vi "rsidr_core_global.vi"() -> ()   [LabVIEW 2015, in "Rohde&Schwarz CMXP NR FR2 Measurement.lvlib"] (continued)
Available Repeated Capabilities:\ninstance: i0, i1, i2, i3, i4, i5, i6, i7, i8, i9, i10, i11, i12, i13, i14, i15, i16, i17, i18, i19, i20, i21, i22, i23, i24, i25, i26, i27, i28, i29, i30, i31, i32\r\n\nRemote-control command(s):\nCONFigure:NRMMw:MEAS<i>:MEValuation:LIMit:QAM64:EVMagnitude"}, {"Level"=5, "Class Only"=FALSE, "Identifier"="RSCMXPNRFR2M_ATTR_MULTI_EVAL_MEASUREMENT_LIMIT_QAM256_EVM", "Descriptive Name"="Multi Eval Measurement Limit QAM256 EVM", "Data Type"=enum."RawString", "Command"="CONF:NRMM:MEAS{instance}:MEV:LIM:QAM256:EVM", "Access"=enum."Read/Write", "Range Table"="", "Read Callback"="", "Write Callback"="", "Range Callback"="", "Check Callback"="", "Rngtable Callback"="", "Coerce Callback"="", "Supported Models"="", "Instrument Options"="", "Check Status Callback"="", "Flags"=0, "Help"="Defines upper limits for the RMS and peak values of the error vector magnitude (EVM) for QAM256.\n\nSyntax:\nCONFigure:NRMMw:MEAS<i>:MEValuation:LIMit:QAM256:EVMagnitude <RMS>, <Peak>\n\n<RMS>\nnumeric | ON | OFF\nValid Values:\n0 % to 100 %\nOFF\nON\n  \n<Peak>\nnumeric | ON | OFF\nValid Values:\n0 % to 100 %\nOFF\nON\n\nAvailable Repeated Capabilities:\ninstance: i0, i1, i2, i3, i4, i5, i6, i7, i8, i9, i10, i11, i12, i13, i14, i15, i16, i17, i18, i19, i20, i21, i22, i23, i24, i25, i26, i27, i28, i29, i30, i31, i32\r\n\nRemote-control command(s):\nCONFigure:NRMMw:MEAS<i>:MEValuation:LIMit:QAM256:EVMagnitude"}, {"Level"=5, "Class Only"=FALSE, "Identifier"="RSCMXPNRFR2M_ATTR_MULTI_EVAL_MEASUREMENT_LIMIT_QAM16_MERR", "Descriptive Name"="Multi Eval Measurement Limit QAM16 MERR", "Data Type"=enum."RawString", "Command"="CONF:NRMM:MEAS{instance}:MEV:LIM:QAM16:MERR", "Access"=enum."Read/Write", "Range Table"="", "Read Callback"="", "Write Callback"="", "Range Callback"="", "Check Callback"="", "Rngtable Callback"="", "Coerce Callback"="", "Supported Models"="", "Instrument Options"="", "Check Status Callback"="", "Flags"=0, "Help"="Defines upper limits for the RMS and peak values of the magnitude error (MERR)  for QAM16.\n\nSyntax:\nCONFigure:NRMMw:MEAS<i>:MEValuation:LIMit:QAM16:MERRor <RMS>, <Peak>\n\n<RMS>\nnumeric | ON | OFF\nValid Values:\n0 % to 100 %\nOFF\nON\n  \n<Peak>\nnumeric | ON | OFF\nValid Values:\n0 % to 100 %\nOFF\nON\n\nAvailable Repeated Capabilities:\ninstance: i0, i1, i2, i3, i4, i5, i6, i7, i8, i9, i10, i11, i12, i13, i14, i15, i16, i17, i18, i19, i20, i21, i22, i23, i24, i25, i26, i27, i28, i29, i30, i31, i32\r\n\nRemote-control command(s):\nCONFigure:NRMMw:MEAS<i>:MEValuation:LIMit:QAM16:MERRor"}, {"Level"=5, "Class Only"=FALSE, "Identifier"="RSCMXPNRFR2M_ATTR_MULTI_EVAL_MEASUREMENT_LIMIT_QAM64_MERR", "Descriptive Name"="Multi Eval Measurement Limit QAM64 MERR", "Data Type"=enum."RawString", "Command"="CONF:NRMM:MEAS{instance}:MEV:LIM:QAM64:MERR", "Access"=enum."Read/Write", "Range Table"="", "Read Callback"="", "Write Callback"="", "Range Callback"="", "Check Callback"="", "Rngtable Callback"="", "Coerce Callback"="", "Supported Models"="", "Instrument Options"="", "Check Status Callback"="", "Flags"=0, "Help"="Defines upper limits for the RMS and peak values of the magnitude error (MERR)  for QAM64.\n\nSyntax:\nCONFigure:NRMMw:MEAS<i>:MEValuation:LIMit:QAM64:MERRor <RMS>, <Peak>\n\n<RMS>\nnumeric | ON | OFF\nValid Values:\n0 % to 100 %\nOFF\nON\n  \n<Peak>\nnumeric | ON | OFF\nValid Values:\n0 % to 100 %\nOFF\nON\n\nAvailable Repeated Capabilities:\ninstance: i0, i1, i2, i3, i4, i5, i6, i7, i8, i9, i10, i11, i12, i13, i14, i15, i16, i17, i18, i19, i20, i21, i22, i23, i24, i25, i26, i27, i28, i29, i30, i31, i32\r\n\nRemote-control command(s):\nCONFigure:NRMMw:MEAS<i>:MEValuation:LIMit:QAM64:MERRor"}, {"Level"=5, "Class Only"=FALSE, "Identifier"="RSCMXPNRFR2M_ATTR_MULTI_EVAL_MEASUREMENT_LIMIT_QAM256_MERR", "Descriptive Name"="Multi Eval Measurement Limit QAM256 MERR", "Data Type"=enum."RawString", "Command"="CONF:NRMM:MEAS{instance}:MEV:LIM:QAM256:MERR", "Access"=enum."Read/Write", "Range Table"="", "Read Callback"="", "Write Callback"="", "Range Callback"="", "Check Callback"="", "Rngtable Callback"="", "Coerce Callback"="", "Supported Models"="", "Instrument Options"="", "Check Status Callback"="", "Flags"=0, "Help"="Defines upper limits for the RMS and peak values of the magnitude error (MERR)  for QAM256.\n\nSyntax:\nCONFigure:NRMMw:MEAS<i>:MEValuation:LIMit:QAM256:MERRor <RMS>, <Peak>\n\n<RMS>\nnumeric | ON | OFF\nValid Values:\n0 % to 100 %\nOFF\nON\n  \n<Peak>\nnumeric | ON | OFF\nValid Values:\n0 % to 100 %\nOFF\nON\n\nAvailable Repeated Capabilities:\ninstance: i0, i1, i2, i3, i4, i5, i6, i7, i8, i9, i10, i11, i12, i13, i14, i15, i16, i17, i18, i19, i20, i21, i22, i23, i24, i25, i26, i27, i28, i29, i30, i31, i32\r\n\nRemote-control command(s):\nCONFigure:NRMMw:MEAS<i>:MEValuation:LIMit:QAM256:MERRor"}, {"Level"=5, "Class Only"=FALSE, "Identifier"="RSCMXPNRFR2M_ATTR_MULTI_EVAL_MEASUREMENT_LIMIT_QAM16_PERR", "Descriptive Name"="Multi Eval Measurement Limit QAM16 PERR", "Data Type"=enum."RawString", "Command"="CONF:NRMM:MEAS{instance}:MEV:LIM:QAM16:PERR", "Access"=enum."Read/Write", "Range Table"="", "Read Callback"="", "Write Callback"="", "Range Callback"="", "Check Callback"="", "Rngtable Callback"="", "Coerce Callback"="", "Supported Models"="", "Instrument Options"="", "Check Status Callback"="", "Flags"=0, "Help"="Defines upper limits for the RMS and peak values of the phase error (PERR)  for QAM16.\n\nSyntax:\nCONFigure:NRMMw:MEAS<i>:MEValuation:LIMit:QAM16:PERRor <RMS>, <Peak>\n\n<RMS>\nnumeric | ON | OFF\nValid Values:\n0 % to 100 %\nOFF\nON\n  \n<Peak>\nnumeric | ON | OFF\nValid Values:\n0 % to 100 %\nOFF\nON\n\nAvailable Repeated Capabilities:\ninstance: i0, i1, i2, i3, i4, i5, i6, i7, i8, i9, i10, i11, i12, i13, i14, i15, i16, i17, i18, i19, i20, i21, i22, i23, i24, i25, i26, i27, i28, i29, i30, i31, i32\r\n\nRemote-control command(s):\nCONFigure:NRMMw:MEAS<i>:MEValuation:LIMit:QAM16:PERRor"}, {"Level"=5, "Class Only"=FALSE, "Identifier"="RSCMXPNRFR2M_ATTR_MULTI_EVAL_MEASUREMENT_LIMIT_QAM64_PERR", "Descriptive Name"="Multi Eval Measurement Limit QAM64 PERR", "Data Type"=enum."RawString", "Command"="CONF:NRMM:MEAS{instance}:MEV:LIM:QAM64:PERR", "Access"=enum."Read/Write", "Range Table"="", "Read Callback"="", "Write Callback"="", "Range Callback"="", "Check Callback"="", "Rngtable Callback"="", "Coerce Callback"="", "Supported Models"="", "Instrument Options"="", "Check Status Callback"="", "Flags"=0, "Help"="Defines upper limits for the RMS and peak values of the phase error (PERR)  for QAM64.\n\nSyntax:\nCONFigure:NRMMw:MEAS<i>:MEValuation:LIMit:QAM64:PERRor <RMS>, <Peak>\n\n<RMS>\nnumeric | ON | OFF\nValid Values:\n0 % to 100 %\nOFF\nON\n  \n<Peak>\nnumeric | ON | OFF\nValid Values:\n0 % to 100 %\nOFF\nON\n\nAvailable Repeated Capabilities:\ninstance: i0, i1, i2, i3, i4, i5, i6, i7, i8, i9, i10, i11, i12, i13, i14, i15, i16, i17, i18, i19, i20, i21, i22, i23, i24, i25, i26, i27, i28, i29, i30, i31, i32\r\n\nRemote-control command(s):\nCONFigure:NRMMw:MEAS<i>:MEValuation:LIMit:QAM64:PERRor"}, {"Level"=5, "Class Only"=FALSE, "Identifier"="RSCMXPNRFR2M_ATTR_MULTI_EVAL_MEASUREMENT_LIMIT_QAM256_PERR", "Descriptive Name"="Multi Eval Measurement Limit QAM256 PERR", "Data Type"=enum."RawString", "Command"="CONF:NRMM:MEAS{instance}:MEV:LIM:QAM256:PERR", "Access"=enum."Read/Write", "Range Table"="", "Read Callback"="", "Write Callback"="", "Range Callback"="", "Check Callback"="", "Rngtable Callback"="", "Coerce Callback"="", "Supported Models"="", "Instrument Options"="", "Check Status Callback"="", "Flags"=0, "Help"="Defines upper limits for the RMS and peak values of the phase error (PERR)  for QAM256.\n\nSyntax:\nCONFigure:NRMMw:MEAS<i>:MEValuation:LIMit:QAM256:PERRor <RMS>, <Peak>\n\n<RMS>\nnumeric | ON | OFF\nValid Values:\n0 % to 100 %\nOFF\nON\n  \n<Peak>\nnumeric | ON | OFF\nValid Values:\n0 % to 100 %\nOFF\nON\n\nAvailable Repeated Capabilities:\ninstance: i0, i1, i2, i3, i4, i5, i6, i7, i8, i9, i10, i11, i12, i13, i14, i15, i16, i17, i18, i19, i20, i21, i22, i23, i24, i25, i26, i27, i28, i29, i30, i31, i32\r\n\nRemote-control command(s):\nCONFigure:NRMMw:MEAS<i>:MEValuation:LIMit:QAM256:PERRor"}, {"Level"=5, "Class Only"=FALSE, "Identifier"="RSCMXPNRFR2M_ATTR_MULTI_EVAL_MEASUREMENT_LIMIT_QAM16_FERR", "Descriptive Name"="Multi Eval Measurement Limit QAM16 FERR", "Data Type"=enum."RawString", "Command"="CONF:NRMM:MEAS{instance}:MEV:LIM:QAM16:FERR", "Access"=enum."Read/Write", "Range Table"="", "Read Callback"="", "Write Callback"="", "Range Callback"="", "Check Callback"="", "Rngtable Callback"="", "Coerce Callback"="", "Supported Models"="", "Instrument Options"="", "Check Status Callback"="", "Flags"=0, "Help"="Defines an upper limit for the carrier frequency error.\n\nSyntax:\nCONFigure:NRMMw:MEAS<i>:MEValuation:LIMit:QAM16:FERRor <FrequencyError>\n\n<FrequencyError>\nnumeric | ON | OFF\nValid Values:\n0 to 1 ppm\nOFF\nON\n\nAvailable Repeated Capabilities:\ninstance: i0, i1, i2, i3, i4, i5, i6, i7, i8, i9, i10, i11, i12, i13, i14, i15, i16, i17, i18, i19, i20, i21, i22, i23, i24, i25, i26, i27, i28, i29, i30, i31, i32\r\n\nRemote-control command(s):\nCONFigure:NRMMw:MEAS<i>:MEValuation:LIMit:QAM16:FERRor"}, {"Level"=5, "Class Only"=FALSE, "Identifier"="RSCMXPNRFR2M_ATTR_MULTI_EVAL_MEASUREMENT_LIMIT_QAM64_FERR", "Descriptive Name"="Multi Eval Measurement Limit QAM64 FERR", "Data Type"=enum."RawString", "Command"="CONF:NRMM:MEAS{instance}:MEV:LIM:QAM64:FERR", "Access"=enum."Read/Write", "Range Table"="", "Read Callback"="", "Write Callback"="", "Range Callback"="", "Check Callback"="", "Rngtable Callback"="", "Coerce Callback"="", "Supported Models"="", "Instrument Options"="", "Check Status Callback"="", "Flags"=0, "Help"="Defines an upper limit for the carrier frequency error.\n\nSyntax:\nCONFigure:NRMMw:MEAS<i>:MEValuation:LIMit:QAM64:FERRor <FrequencyError>\n\n<FrequencyError>\nnumeric | ON | OFF\nValid Values:\n0 to 1 ppm\nOFF\nON\n\nAvailable Repeated Capabilities:\ninstance: i0, i1, i2, i3, i4, i5, i6, i7, i8, i9, i10, i11, i12, i13, i14, i15, i16, i17, i18, i19, i20, i21, i22, i23, i24, i25, i26, i27, i28, i29, i30, i31, i32\r\n\nRemote-control command(s):\nCONFigure:NRMMw:MEAS<i>:MEValuation:LIMit:QAM64:FERRor"}, {"Level"=5, "Class Only"=FALSE, "Identifier"="RSCMXPNRFR2M_ATTR_MULTI_EVAL_MEASUREMENT_LIMIT_QAM256_FERR", "Descriptive Name"="Multi Eval Measurement Limit QAM256 FERR", "Data Type"=enum."RawString", "Command"="CONF:NRMM:MEAS{instance}:MEV:LIM:QAM256:FERR", "Access"=enum."Read/Write", "Range Table"="", "Read Callback"="", "Write Callback"="", "Range Callback"="", "Check Callback"="", "Rngtable Callback"="", "Coerce Callback"="", "Supported Models"="", "Instrument Options"="", "Check Status Callback"="", "Flags"=0, "Help"="Defines an upper limit for the carrier frequency error.\n\nSyntax:\nCONFigure:NRMMw:MEAS<i>:MEValuation:LIMit:QAM256:FERRor <FrequencyError>\n\n<FrequencyError>\nnumeric | ON | OFF\nValid Values:\n0 to 1 ppm\nOFF\nON\n\nAvailable Repeated Capabilities:\ninstance: i0, i1, i2, i3, i4, i5, i6, i7, i8, i9, i10, i11, i12, i13, i14, i15, i16, i17, i18, i19, i20, i21, i22, i23, i24, i25, i26, i27, i28, i29, i30, i31, i32\r\n\nRemote-control command(s):\nCONFigure:NRMMw:MEAS<i>:MEValuation:LIMit:QAM256:FERRor"}, {"Level"=5, "Class Only"=FALSE, "Identifier"="RSCMXPNRFR2M_ATTR_MULTI_EVAL_MEASUREMENT_LIMIT_QAM16_IQ_OFFSET", "Descriptive Name"="Multi Eval Measurement Limit QAM16 IQ Offset", "Data Type"=enum."RawString", "Command"="CONF:NRMM:MEAS{instance}:MEV:LIM:QAM16:IQOF", "Access"=enum."Read/Write", "Range Table"="", "Read Callback"="", "Write Callback"="", "Range Callback"="", "Check Callback"="", "Rngtable Callback"="", "Coerce Callback"="", "Supported Models"="", "Instrument Options"="", "Check Status Callback"="", "Flags"=0, "Help"="Defines upper limits for the I/Q origin offset (QAM16 modulation). Two different I/Q origin offset limits can be set for two TX power ranges.\n\nSyntax:\nCONFigure:NRMMw:MEAS<i>:MEValuation:LIMit:QAM16:IQOFfset <Enable>, <Offset0>, <Offset1>\n\n<Enable>\nValid Values:\nOFF: disables the limit check\nON: enables the limit check\n\n<Offset0>\nI/Q origin offset limit for TX power > 0 dBm\nnumeric\nValid Values: -256 dBc to 256 dBc\n\n<Offset1>\nI/Q origin offset limit for TX power  0 dBm\nnumeric\nValid Values: -256 dBc to 256 dBc\n\nAvailable Repeated Capabilities:\ninstance: i0, i1, i2, i3, i4, i5, i6, i7, i8, i9, i10, i11, i12, i13, i14, i15, i16, i17, i18, i19, i20, i21, i22, i23, i24, i25, i26, i27, i28, i29, i30, i31, i32\r\n\nRemote-control command(s):\nCONFigure:NRMMw:MEAS<i>:MEValuation:LIMit:QAM16:IQOFfset"}, {"Level"=5, "Class Only"=FALSE, "Identifier"="RSCMXPNRFR2M_ATTR_MULTI_EVAL_MEASUREMENT_LIMIT_QAM64_IQ_OFFSET", "Descriptive Name"="Multi Eval Measurement Limit QAM64 IQ Offset", "Data Type"=enum."RawString", "Command"="CONF:NRMM:MEAS{instance}:MEV:LIM:QAM64:IQOF", "Access"=enum."Read/Write", "Range Table"="", "Read Callback"="", "Write Callback"="", "Range Callback"="", "Check Callback"="", "Rngtable Callback"="", "Coerce Callback"="", "Supported Models"="", "Instrument Options"="", "Check Status Callback"="", "Flags"=0, "Help"="Defines upper limits for the I/Q origin offset (QAM64 modulation). Two different I/Q origin offset limits can be set for two TX power ranges.\n\nSyntax:\nCONFigure:NRMMw:MEAS<i>:MEValuation:LIMit:QAM64:IQOFfset <Enable>, <Offset0>, <Offset1>\n\n<Enable>\nValid Values:\nOFF: disables the limit check\nON: enables the limit check\n\n<Offset0>\nI/Q origin offset limit for TX power > 0 dBm\nnumeric\nValid Values: -256 dBc to 256 dBc\n\n<Offset1>\nI/Q origin offset limit for TX power  0 dBm\nnumeric\nValid Values: -256 dBc to 256 dBc\n\nAvailable Repeated Capabilities:\ninstance: i0, i1, i2, i3, i4, i5, i6, i7, i8, i9, i10, i11, i12, i13, i14, i15, i16, i17, i18, i19, i20, i21, i22, i23, i24, i25, i26, i27, i28, i29, i30, i31, i32\r\n\nRemote-control command(s):\nCONFigure:NRMMw:MEAS<i>:MEValuation:LIMit:QAM64:IQOFfset"}, {"Level"=5, "Class Only"=FALSE, "Identifier"="RSCMXPNRFR2M_ATTR_MULTI_EVAL_MEASUREMENT_LIMIT_QAM256_IQ_OFFSET", "Descriptive Name"="Multi Eval Measurement Limit QAM256 IQ Offset", "Data Type"=enum."RawString", "Command"="CONF:NRMM:MEAS{instance}:MEV:LIM:QAM256:IQOF", "Access"=enum."Read/Write", "Range Table"="", "Read Callback"="", "Write Callback"="", "Range Callback"="", "Check Callback"="", "Rngtable Callback"="", "Coerce Callback"="", "Supported Models"="", "Instrument Options"="", "Check Status Callback"="", "Flags"=0, "Help"="Defines upper limits for the I/Q origin offset (QAM256 modulation). Two different I/Q origin offset limits can be set for two TX power ranges.\n\nSyntax:\nCONFigure:NRMMw:MEAS<i>:MEValuation:LIMit:QAM256:IQOFfset <Enable>, <Offset0>, <Offset1>\n\n<Enable>\nValid Values:\nOFF: disables the limit check\nON: enables the limit check\n\n<Offset0>\nI/Q origin offset limit for TX power > 0 dBm\nnumeric\nValid Values: -256 dBc to 256 dBc\n\n<Offset1>\nI/Q origin offset limit for TX power  0 dBm\nnumeric\nValid Values: -256 dBc to 256 dBc\n\nAvailable Repeated Capabilities:\ninstance: i0, i1, i2, i3, i4, i5, i6, i7, i8, i9, i10, i11, i12, i13, i14, i15, i16, i17, i18, i19, i20, i21, i22, i23, i24, i25, i26, i27, i28, i29, i30, i31, i32\r\n\nRemote-control command(s):\nCONFigure:NRMMw:MEAS<i>:MEValuation:LIMit:QAM256:IQOFfset"}, {"Level"=5, "Class Only"=FALSE, "Identifier"="RSCMXPNRFR2M_ATTR_MULTI_EVAL_MEASUREMENT_LIMIT_QAM16_INBAND_EMISSION", "Descriptive Name"="Multi Eval Measurement Limit QAM16 Inband Emission", "Data Type"=enum."RawString", "Command"="CONF:NRMM:MEAS{instance}:MEV:LIM:QAM16:IBE", "Access"=enum."Read/Write", "Range Table"="", "Read Callback"="", "Write Callback"="", "Range Callback"="", "Check Callback"="", "Rngtable Callback"="", "Coerce Callback"="", "Supported Models"="", "Instrument Options"="", "Check Status Callback"="", "Flags"=0, "Help"="Defines parameters used for calculation of an upper limit for the inband emission (QAM16 modulation).\n\nSyntax:\nCONFigure:NRMMw:MEAS<i>:MEValuation:LIMit:QAM16:IQOFfset <Enable>, <Offset0>, <Offset1>\n\n<Enable>\nValid Values:\nOFF: disables the limit check\nON: enables the limit check\n\n<Minimum>\nnumeric\nValid Values: -256 dB to 256 dB\n\n<EVM>\nnumeric\nValid Values: 0 % to 100 %\n\n<RBPower>\nnumeric\nValid Values: -256 dBm to 256 dBm\n\n<IQImageLesser>\nIQ image for low TX power range\nnumeric\nValid Values: -256 dB to 256 dB\n \n<IQImageGreater>\nIQ image for high TX power range\nnumeric\nValid Values: -256 dB  to  256 dB\n\nAvailable Repeated Capabilities:\ninstance: i0, i1, i2, i3, i4, i5, i6, i7, i8, i9, i10, i11, i12, i13, i14, i15, i16, i17, i18, i19, i20, i21, i22, i23, i24, i25, i26, i27, i28, i29, i30, i31, i32\r\n\nRemote-control command(s):\nCONFigure:NRMMw:MEAS<i>:MEValuation:LIMit:QAM16:IBE"}, {"Level"=5, "Class Only"=FALSE, "Identifier"="RSCMXPNRFR2M_ATTR_MULTI_EVAL_MEASUREMENT_LIMIT_QAM64_INBAND_EMISSION", "Descriptive Name"="Multi Eval Measurement Limit QAM64 Inband Emission", "Data Type"=enum."RawString", "Command"="CONF:NRMM:MEAS{instance}:MEV:LIM:QAM64:IBE", "Access"=enum."Read/Write", "Range Table"="", "Read Callback"="", "Write Callback"="", "Range Callback"="", "Check Callback"="", "Rngtable Callback"="", "Coerce Callback"="", "Supported Models"="", "Instrument Options"="", "Check Status Callback"="", "Flags"=0, "Help"="Defines parameters used for calculation of an upper limit for the inband emission (QAM64 modulation).\n\nSyntax:\nCONFigure:NRMMw:MEAS<i>:MEValuation:LIMit:QAM64:IQOFfset <Enable>, <Offset0>, <Offset1>\n\n<Enable>\nValid Values:\nOFF: disables the limit check\nON: enables the limit check\n\n<Minimum>\nnumeric\nValid Values: -256 dB to 256 dB\n\n<EVM>\nnumeric\nValid Values: 0 % to 100 %\n\n<RBPower>\nnumeric\nValid Values: -256 dBm to 256 dBm\n\n<IQImageLesser>\nIQ image for low TX power range\nnumeric\nValid Values: -256 dB to 256 dB\n \n<IQImageGreater>\nIQ image for high TX power range\nnumeric\nValid Values: -256 dB  to  256 dB\n\nAvailable Repeated Capabilities:\ninstance: i0, i1, i2, i3, i4, i5, i6, i7, i8, i9, i10, i11, i12, i13, i14, i15, i16, i17, i18, i19, i20, i21, i22, i23, i24, i25, i26, i27, i28, i29, i30, i31, i32\r\n\nRemote-control command(s):\nCONFigure:NRMMw:MEAS<i>:MEValuation:LIMit:QAM64:IBE"}, {"Level"=5, "Class Only"=FALSE, "Identifier"="RSCMXPNRFR2M_ATTR_MULTI_EVAL_MEASUREMENT_LIMIT_QAM256_INBAND_EMISSION", "Descriptive Name"="Multi Eval Measurement Limit QAM256 Inband Emission", "Data Type"=enum."RawString", "Command"="CONF:NRMM:MEAS{instance}:MEV:LIM:QAM256:IBE", "Access"=enum."Read/Write", "Range Table"="", "Read Callback"="", "Write Callback"="", "Range Callback"="", "Check Callback"="", "Rngtable Callback"="", "Coerce Callback"="", "Supported Models"="", "Instrument Options"="", "Check Status Callback"="", "Flags"=0, "Help"="Defines parameters used for calculation of an upper limit for the inband emission (QAM256 modulation).\n\nSyntax:\nCONFigure:NRMMw:MEAS<i>:MEValuation:LIMit:QAM256:IQOFfset <Enable>, <Offset0>, <Offset1>\n\n<Enable>\nValid Values:\nOFF: disables the limit check\nON: enables the limit check\n\n<Minimum>\nnumeric\nValid Values: -256 dB to 256 dB\n\n<EVM>\nnumeric\nValid Values: 0 % to 100 %\n\n<RBPower>\nnumeric\nValid Values: -256 dBm to 256 dBm\n\n<IQImageLesser>\nIQ image for low TX power range\nnumeric\nValid Values: -256 dB to 256 dB\n \n<IQImageGreater>\nIQ image for high TX power range\nnumeric\nValid Values: -256 dB  to  256 dB\n\nAvailable Repeated Capabilities:\ninstance: i0, i1, i2, i3, i4, i5, i6, i7, i8, i9, i10, i11, i12, i13, i14, i15, i16, i17, i18, i19, i20, i21, i22, i23, i24, i25, i26, i27, i28, i29, i30, i31, i32\r\n\nRemote-control command(s):\nCONFigure:NRMMw:MEAS<i>:MEValuation:LIMit:QAM256:IBE"}, {"Level"=5, "Class Only"=FALSE, "Identifier"="RSCMXPNRFR2M_ATTR_MULTI_EVAL_MEASUREMENT_LIMIT_QAM16_INBAND_EMISSION_IQ_OFFSET", "Descriptive Name"="Multi Eval Measurement Limit QAM16 Inband Emission IQ Offset", "Data Type"=enum."RawString", "Command"="CONF:NRMM:MEAS{instance}:MEV:LIM:QAM16:IBE:IQOF", "Access"=enum."Read/Write", "Range Table"="", "Read Callback"="", "Write Callback"="", "Range Callback"="", "Check Callback"="", "Rngtable Callback"="", "Coerce Callback"="", "Supported Models"="", "Instrument Options"="", "Check Status Callback"="", "Flags"=0, "Help"="Defines I/Q origin offset values used for calculation of an upper limit for the inband emission, for QAM16 modulation. Two different values can be set for two TX power ranges.\n\nSyntax:\nCONFigure:NRMMw:MEAS<i>:MEValuation:LIMit:QAM16:IBE:IQOFfset <Offset0>, <Offset1>\n\n<Offset0>\nI/Q origin offset limit for TX power > 0 dBm\nnumeric\nValid Values: -256 dBc to 256 dBc\n\n<Offset1>\nI/Q origin offset limit for TX power  0 dBm\nnumeric\nValid Values: -256 dBc to 256 dBc\n\nAvailable Repeated Capabilities:\ninstance: i0, i1, i2, i3, i4, i5, i6, i7, i8, i9, i10, i11, i12, i13, i14, i15, i16, i17, i18, i19, i20, i21, i22, i23, i24, i25, i26, i27, i28, i29, i30, i31, i32\r\n\nRemote-control command(s):\nCONFigure:NRMMw:MEAS<i>:MEValuation:LIMit:QAM16:IBE:IQOFfset"}, {"Level"=5, "Class Only"=FALSE, "Identifier"="RSCMXPNRFR2M_ATTR_MULTI_EVAL_MEASUREMENT_LIMIT_QAM64_INBAND_EMISSION_IQ_OFFSET", "Descriptive Name"="Multi Eval Measurement Limit QAM64 Inband Emission IQ Offset", "Data Type"=enum."RawString", "Command"="CONF:NRMM:MEAS{instance}:MEV:LIM:QAM64:IBE:IQOF", "Access"=enum."Read/Write", "Range Table"="", "Read Callback"="", "Write Callback"="", "Range Callback"="", "Check Callback"="", "Rngtable Callback"="", "Coerce Callback"="", "Supported Models"="", "Instrument Options"="", "Check Status Callback"="", "Flags"=0, "Help"="Defines I/Q origin offset values used for calculation of an upper limit for the inband emission, for QAM64 modulation. Two different values can be set for two TX power ranges.\n\nSyntax:\nCONFigure:NRMMw:MEAS<i>:MEValuation:LIMit:QAM64:IBE:IQOFfset <Offset0>, <Offset1>\n\n<Offset0>\nI/Q origin offset limit for TX power > 0 dBm\nnumeric\nValid Values: -256 dBc to 256 dBc\n\n<Offset1>\nI/Q origin offset limit for TX power  0 dBm\nnumeric\nValid Values: -256 dBc to 256 dBc\n\nAvailable Repeated Capabilities:\ninstance: i0, i1, i2, i3, i4, i5, i6, i7, i8, i9, i10, i11, i12, i13, i14, i15, i16, i17, i18, i19, i20, i21, i22, i23, i24, i25, i26, i27, i28, i29, i30, i31, i32\r\n\nRemote-control command(s):\nCONFigure:NRMMw:MEAS<i>:MEValuation:LIMit:QAM64:IBE:IQOFfset"}, {"Level"=5, "Class Only"=FALSE, "Identifier"="RSCMXPNRFR2M_ATTR_MULTI_EVAL_MEASUREMENT_LIMIT_QAM256_INBAND_EMISSION_IQ_OFFSET", "Descriptive Name"="Multi Eval Measurement Limit QAM256 Inband Emission IQ Offset", "Data Type"=enum."RawString", "Command"="CONF:NRMM:MEAS{instance}:MEV:LIM:QAM256:IBE:IQOF", "Access"=enum."Read/Write", "Range Table"="", "Read Callback"="", "Write Callback"="", "Range Callback"="", "Check Callback"="", "Rngtable Callback"="", "Coerce Callback"="", "Supported Models"="", "Instrument Options"="", "Check Status Callback"="", "Flags"=0, "Help"="Defines I/Q origin offset values used for calculation of an upper limit for the inband emission, for QAM256 modulation. Two different values can be set for two TX power ranges.\n\nSyntax:\nCONFigure:NRMMw:MEAS<i>:MEValuation:LIMit:QAM256:IBE:IQOFfset <Offset0>, <Offset1>\n\n<Offset0>\nI/Q origin offset limit for TX power > 0 dBm\nnumeric\nValid Values: -256 dBc to 256 dBc\n\n<Offset1>\nI/Q origin offset limit for TX power  0 dBm\nnumeric\nValid Values: -256 dBc to 256 dBc\n\nAvailable Repeated Capabilities:\ninstance: i0, i1, i2, i3, i4, i5, i6, i7, i8, i9, i10, i11, i12, i13, i14, i15, i16, i17, i18, i19, i20, i21, i22, i23, i24, i25, i26, i27, i28, i29, i30, i31, i32\r\n\nRemote-control command(s):\nCONFigure:NRMMw:MEAS<i>:MEValuation:LIMit:QAM256:IBE:IQOFfset"}, {"Level"=5, "Class Only"=FALSE, "Identifier"="RSCMXPNRFR2M_ATTR_MULTI_EVAL_MEASUREMENT_LIMIT_QAM16_EQUALIZER_SPECTRUM_FLATNESS", "Descriptive Name"="Multi Eval Measurement Limit QAM16 Equalizer Spectrum Flatness", "Data Type"=enum."RawString", "Command"="CONF:NRMM:MEAS{instance}:MEV:LIM:QAM16:ESFL", "Access"=enum."Read/Write", "Range Table"="", "Read Callback"="", "Write Callback"="", "Range Callback"="", "Check Callback"="", "Rngtable Callback"="", "Coerce Callback"="", "Supported Models"="", "Instrument Options"="", "Check Status Callback"="", "Flags"=0, "Help"="Defines limits for the equalizer spectrum flatness (QAM16 modulation).\n\nSyntax:\nCONFigure:NRMMw:MEAS<i>:MEValuation:LIMit:QAM16:IQOFfset <Enable>, <Offset0>, <Offset1>\n\n<Enable>\nValid Values:\nOFF: disables the limit check\nON: enables the limit check\n\n<Range1>\nUpper limit for max(range 1) - min(range 1)\nnumeric\nValid Values: -256 dBpp to 256 dBpp \n\n<Range2>\nUpper limit for max(range 2) - min(range 2)\nnumeric\nValid Values: -256 dBpp to 256 dBpp \n\n<Max1Min2>\nUpper limit for max(range 1) - min(range 2)\nnumeric\nValid Values: -256 dB to 256 dB \n\n<Max2Min1>\nUpper limit for max(range 2) - min(range 1)\nnumeric\nValid Values: -256 dB to 256 dB\n\nAvailable Repeated Capabilities:\ninstance: i0, i1, i2, i3, i4, i5, i6, i7, i8, i9, i10, i11, i12, i13, i14, i15, i16, i17, i18, i19, i20, i21, i22, i23, i24, i25, i26, i27, i28, i29, i30, i31, i32\r\n\nRemote-control command(s):\nCONFigure:NRMMw:MEAS<i>:MEValuation:LIMit:QAM16:ESFLatness"}, {"Level"=5, "Class Only"=FALSE, "Identifier"="RSCMXPNRFR2M_ATTR_MULTI_EVAL_MEASUREMENT_LIMIT_QAM64_EQUALIZER_SPECTRUM_FLATNESS", "Descriptive Name"="Multi Eval Measurement Limit QAM64 Equalizer Spectrum Flatness", "Data Type"=enum."RawString", "Command"="CONF:NRMM:MEAS{instance}:MEV:LIM:QAM64:ESFL", "Access"=enum."Read/Write", "Range Table"="", "Read Callback"="", "Write Callback"="", "Range Callback"="", "Check Callback"="", "Rngtable Callback"="", "Coerce Callback"="", "Supported Models"="", "Instrument Options"="", "Check Status Callback"="", "Flags"=0, "Help"="Defines limits for the equalizer spectrum flatness (QAM64 modulation).\n\nSyntax:\nCONFigure:NRMMw:MEAS<i>:MEValuation:LIMit:QAM64:IQOFfset <Enable>, <Offset0>, <Offset1>\n\n<Enable>\nValid Values:\nOFF: disables the limit check\nON: enables the limit check\n\n<Range1>\nUpper limit for max(range 1) - min(range 1)\nnumeric\nValid Values: -256 dBpp to 256 dBpp \n\n<Range2>\nUpper limit for max(range 2) - min(range 2)\nnumeric\nValid Values: -256 dBpp to 256 dBpp \n\n<Max1Min2>\nUpper limit for max(range 1) - min(range 2)\nnumeric\nValid Values: -256 dB to 256 dB \n\n<Max2Min1>\nUpper limit for max(range 2) - min(range 1)\nnumeric\nValid Values: -256 dB to 256 dB\n\nAvailable Repeated Capabilities:\ninstance: i0, i1, i2, i3, i4, i5, i6, i7, i8, i9, i10, i11, i12, i13, i14, i15, i16, i17, i18, i19, i20, i21, i22, i23, i24, i25, i26, i27, i28, i29, i30, i31, i32\r\n\nRemote-control command(s):\nCONFigure:NRMMw:MEAS<i>:MEValuation:LIMit:QAM64:ESFLatness"}, {"Level"=5, "Class Only"=FALSE, "Identifier"="RSCMXPNRFR2M_ATTR_MULTI_EVAL_MEASUREMENT_LIMIT_QAM256_EQUALIZER_SPECTRUM_FLATNESS", "Descriptive Name"="Multi Eval Measurement Limit QAM256 Equalizer Spectrum Flatness", "Data Type"=enum."RawString", "Command"="CONF:NRMM:MEAS{instance}:MEV:LIM:QAM256:ESFL", "Access"=enum."Read/Write", "Range Table"="", "Read Callback"="", "Write Callback"="", "Range Callback"="", "Check Callback"="", "Rngtable Callback"="", "Coerce Callback"="", "Supported Models"="", "Instrument Options"="", "Check Status Callback"="", "Flags"=0, "Help"="Defines limits for the equalizer spectrum flatness (QAM256 modulation).\n\nSyntax:\nCONFigure:NRMMw:MEAS<i>:MEValuation:LIMit:QAM256:IQOFfset <Enable>, <Offset0>, <Offset1>\n\n<Enable>\nValid Values:\nOFF: disables the limit check\nON: enables the limit check\n\n<Range1>\nUpper limit for max(range 1) - min(range 1)\nnumeric\nValid Values: -256 dBpp to 256 dBpp \n\n<Range2>\nUpper limit for max(range 2) - min(range 2)\nnumeric\nValid Values: -256 dBpp to 256 dBpp \n\n<Max1Min2>\nUpper limit for max(range 1) - min(range 2)\nnumeric\nValid Values: -256 dB to 256 dB \n\n<Max2Min1>\nUpper limit for max(range 2) - min(range 1)\nnumeric\nValid Values: -256 dB to 256 dB\n\nAvailable Repeated Capabilities:\ninstance: i0, i1, i2, i3, i4, i5, i6, i7, i8, i9, i10, i11, i12, i13, i14, i15, i16, i17, i18, i19, i20, i21, i22, i23, i24, i25, i26, i27, i28, i29, i30, i31, i32\r\n\nRemote-control command(s):\nCONFigure:NRMMw:MEAS<i>:MEValuation:LIMit:QAM256:ESFLatness"}, {"Level"=3, "Class Only"=TRUE, "Identifier"="", "Descriptive Name"="Spectrum", "Data Type"=enum."ViInt32", "Command"="", "Access"=enum."Read Only", "Range Table"="", "Read Callback"="", "Write Callback"="", "Range Callback"="", "Check Callback"="", "Rngtable Callback"="", "Coerce Callback"="", "Supported Models"="", "Instrument Options"="", "Check Status Callback"="", "Flags"=0, "Help"="Spectrum limits definition."}, {"Level"=4, "Class Only"=FALSE, "Identifier"="RSCMXPNRFR2M_ATTR_MULTI_EVAL_MEASUREMENT_LIMIT_OBW_ENABLED", "Descriptive Name"="Multi Eval Measurement Limit OBW Enabled", "Data Type"=enum."ViBoolean", "Command"="CONF:NRMM:MEAS{instance}:MEV:LIM:SEM:OBWL:CBAN{Bandwidth}", "Access"=enum."Write Only", "Range Table"="", "Read Callback"="", "Write Callback"="", "Range Callback"="", "Check Callback"="", "Rngtable Callback"="", "Coerce Callback"="", "Supported Models"="", "Instrument Options"="", "Check Status Callback"="", "Flags"=0, "Help"="Enables/disables an upper limit for the occupied bandwidth, depending on the channel bandwidth.\n\nAvailable Repeated Capabilities:\ninstance: i0, i1, i2, i3, i4, i5, i6, i7, i8, i9, i10, i11, i12, i13, i14, i15, i16, i17, i18, i19, i20, i21, i22, i23, i24, i25, i26, i27, i28, i29, i30, i31, i32\r\nBandwidth: BW50, BW100, BW200, BW400\r\n\nRemote-control command(s):\nCONFigure:NRMMw:MEAS<i>:MEValuation:LIMit:SEMask:OBWLimit:CBANdwidth<bw>"}, {"Level"=4, "Class Only"=FALSE, "Identifier"="RSCMXPNRFR2M_ATTR_MULTI_EVAL_MEASUREMENT_LIMIT_OBW", "Descriptive Name"="Multi Eval Measurement Limit OBW", "Data Type"=enum."ViReal64", "Command"="CONF:NRMM:MEAS{instance}:MEV:LIM:SEM:OBWL:CBAN{Bandwidth}", "Access"=enum."Read/Write", "Range Table"="rsCmxpNrFr2M_rngOBWLimit", "Read Callback"="", "Write Callback"="", "Range Callback"="", "Check Callback"="", "Rngtable Callback"="", "Coerce Callback"="", "Supported Models"="", "Instrument Options"="", "Check Status Callback"="", "Flags"=0, "Help"="Defines an upper limit for the occupied bandwidth, depending on the channel bandwidth.\n\nAvailable Repeated Capabilities:\ninstance: i0, i1, i2, i3, i4, i5, i6, i7, i8, i9, i10, i11, i12, i13, i14, i15, i16, i17, i18, i19, i20, i21, i22, i23, i24, i25, i26, i27, i28, i29, i30, i31, i32\r\nBandwidth: BW50, BW100, BW200, BW400\r\n\nRemote-control command(s):\nCONFigure:NRMMw:MEAS<i>:MEValuation:LIMit:SEMask:OBWLimit:CBANdwidth<bw>"}, {"Level"=4, "Class Only"=FALSE, "Identifier"="RSCMXPNRFR2M_ATTR_MULTI_EVAL_MEASUREMENT_LIMIT_EMISSION_MASK", "Descriptive Name"="Multi Eval Measurement Limit Emission Mask", "Data Type"=enum."RawString", "Command"="CONF:NRMM:MEAS{instance}:MEV:LIM:SEM:AREA{Area}:CBAN{Bandwidth}", "Access"=enum."Read/Write", "Range Table"="", "Read Callback"="", "Write Callback"="", "Range Callback"="", "Check Callback"="", "Rngtable Callback"="", "Coerce Callback"="", "Supported Models"="", "Instrument Options"="", "Check Status Callback"="", "Flags"=0, "Help"="Defines general requirements for the emission mask area number <area>. The activation state, the area borders, an upper limit and the resolution bandwidth must be specified.\nThe emission mask applies to the channel bandwidth <bw>.\n\nSyntax:\nCONFigure:NRMMw:MEAS<i>:MEValuation:LIMit:SEMask:AREA<area>:CBANdwidth<bw> <Enable>, <FrequencyStart>, <FrequencyEnd>, <Level>, <RBW>\n\n<bw>\nChannel bandwidth in MHz\nValid Values: 50, 100, 200, 400\n \n<area>\nNumber of the emission mask area\nValid Values: 1 to 12\n\n<Enable>\nValid Values:\nOFF: disables the check of these requirements\nON: enables the check of these requirements\n \n<FrequencyStart>\nStart frequency of the area, relative to the edges of the channel bandwidth\nnumeric\nValid Values: 0 MHz to 405 MHz (less, depending on <bw>) \n \n<FrequencyEnd>\nStop frequency of the area, relative to the edges of the channel bandwidth\nnumeric\nValid Values: 0 MHz to 405 MHz (less, depending on <bw>)\n\n<Level>\nUpper limit for the area\nnumeric\nValid Values: -256 dBm to 256 dBm\n\n<RBW>\nResolution bandwidth to be used for the area (1 MHz)\nValid Values: M1\n\nAvailable Repeated Capabilities:\ninstance: i0, i1, i2, i3, i4, i5, i6, i7, i8, i9, i10, i11, i12, i13, i14, i15, i16, i17, i18, i19, i20, i21, i22, i23, i24, i25, i26, i27, i28, i29, i30, i31, i32\r\nArea: a1, a2, a3, a4, a5, a6, a7, a8, a9, a10, a11, a12\r\nBandwidth: BW50, BW100, BW200, BW400\r\n\nRemote-control command(s):\nCONFigure:NRMMw:MEAS<i>:MEValuation:LIMit:SEMask:AREA<area>:CBANdwidth<bw>"}, {"Level"=4, "Class Only"=FALSE, "Identifier"="RSCMXPNRFR2M_ATTR_MULTI_EVAL_MEASUREMENT_LIMIT_EMISSION_MASK_TEST_TOLERANCE", "Descriptive Name"="Multi Eval Measurement Limit Emission Mask Test Tolerance", "Data Type"=enum."RawString", "Command"="CONF:NRMM:MEAS{instance}:MEV:LIM:SEM:ATT", "Access"=enum."Read/Write", "Range Table"="", "Read Callback"="", "Write Callback"="", "Range Callback"="", "Check Callback"="", "Rngtable Callback"="", "Coerce Callback"="", "Supported Models"="", "Instrument Options"="", "Check Status Callback"="", "Flags"=0, "Help"="Defines the test tolerance for spectrum emission masks, depending on the carrier frequency.\n\nSyntax:\nCONFigure:NRMMw:MEAS<i>:MEValuation:LIMit:SEMask:ATTolerance <Tol23_30>, <Tol30_40>\n\n<Tol23_30>\nTest tolerance for carrier frequencies >= 23.45 GHz and <= 32.125 GHz\nnumeric\nValid Values: -10 dB to 10 dB\n \n<Tol30_40>\nTest tolerance for carrier frequencies > 32.125 GHz and <= 40.8 GHz\nnumeric\nValid Values: -10 dB to 10 dB\n\nAvailable Repeated Capabilities:\ninstance: i0, i1, i2, i3, i4, i5, i6, i7, i8, i9, i10, i11, i12, i13, i14, i15, i16, i17, i18, i19, i20, i21, i22, i23, i24, i25, i26, i27, i28, i29, i30, i31, i32\r\n\nRemote-control command(s):\nCONFigure:NRMMw:MEAS<i>:MEValuation:LIMit:SEMask:ATTolerance"}, {"Level"=4, "Class Only"=FALSE, "Identifier"="RSCMXPNRFR2M_ATTR_MULTI_EVAL_MEASUREMENT_LIMIT_ACLR", "Descriptive Name"="Multi Eval Measurement Limit ACLR", "Data Type"=enum."RawString", "Command"="CONF:NRMM:MEAS{instance}:MEV:LIM:ACLR:NR:CBAN{Bandwidth}:BLIM{LimitBand}", "Access"=enum."Read/Write", "Range Table"="", "Read Callback"="", "Write Callback"="", "Range Callback"="", "Check Callback"="", "Rngtable Callback"="", "Coerce Callback"="", "Supported Models"="", "Instrument Options"="", "Check Status Callback"="", "Flags"=0, "Help"="Defines relative and absolute limits for the ACLR measured in an adjacent NR channel. The settings are defined separately for each channel bandwidth.\n\nSyntax:\nCONFigure:NRMMw:MEAS<i>:MEValuation:LIMit:ACLR:NR:CBANdwidth<bw>:BLIMits<n> <RelativeLevel>, <AbsoluteLevel>\n\n<bw>\nChannel bandwidth in MHz\nValid Values: 50, 100, 200, 400\n \n<n>\nBand\nValid Values:\n1 - band n257, n258, n261\n2 - bands n260\n \n<RelativeLevel>\nRelative lower ACLR limit without test tolerance\nnumeric | ON | OFF\nValid Values: -256 dB to 256 dB\nON | OFF enables or disables the limit check.\n\n<AbsoluteLevel>\n numeric | ON | OFF\nValid Values: -256 dBm to 256 dBm\nON | OFF enables or disables the limit check.\n\nAvailable Repeated Capabilities:\ninstance: i0, i1, i2, i3, i4, i5, i6, i7, i8, i9, i10, i11, i12, i13, i14, i15, i16, i17, i18, i19, i20, i21, i22, i23, i24, i25, i26, i27, i28, i29, i30, i31, i32\r\nBandwidth: BW50, BW100, BW200, BW400\r\nLimitBand: b1, b2\r\n\nRemote-control command(s):\nCONFigure:NRMMw:MEAS<i>:MEValuation:LIMit:ACLR:NR:CBANdwidth<bw>:BLIMits<n>"}, {"Level"=4, "Class Only"=FALSE, "Identifier"="RSCMXPNRFR2M_ATTR_MULTI_EVAL_MEASUREMENT_LIMIT_ACLR_TEST_TOLERANCE", "Descriptive Name"="Multi Eval Measurement Limit ACLR Test Tolerance", "Data Type"=enum."RawString", "Command"="CONF:NRMM:MEAS{instance}:MEV:LIM:ACLR:ATT", "Access"=enum."Read/Write", "Range Table"="", "Read Callback"="", "Write Callback"="", "Range Callback"="", "Check Callback"="", "Rngtable Callback"="", "Coerce Callback"="", "Supported Models"="", "Instrument Options"="", "Check Status Callback"="", "Flags"=0, "Help"="Defines the test tolerance for relative ACLR limits, depending on the carrier frequency.\n\nSyntax:\nCONFigure:NRMMw:MEAS<i>:MEValuation:LIMit:ACLR:ATTolerance <Tol23_30>, <Tol30_40>\n \n<Tol23_30>\nTest tolerance for carrier frequencies >= 23.45 GHz and <= 30.3 GHz\nnumeric\nValid Values: -10 dB to 10 dB\n \n<Tol30_40>\nTest tolerance for carrier frequencies > 30.3 GHz and <= 40.8 GHz\nnumeric\nValid Values: -10 dB to 10 dB\n\nAvailable Repeated Capabilities:\ninstance: i0, i1, i2, i3, i4, i5, i6, i7, i8, i9, i10, i11, i12, i13, i14, i15, i16, i17, i18, i19, i20, i21, i22, i23, i24, i25, i26, i27, i28, i29, i30, i31, i32\r\n\nRemote-control command(s):\nCONFigure:NRMMw:MEAS<i>:MEValuation:LIMit:ACLR:ATTolerance"}, {"Level"=2, "Class Only"=TRUE, "Identifier"="", "Descriptive Name"="Results", "Data Type"=enum."ViInt32", "Command"="", "Access"=enum."Read Only", "Range Table"="", "Read Callback"="", "Write Callback"="", "Range Callback"="", "Check Callback"="", "Rngtable Callback"="", "Coerce Callback"="", "Supported Models"="", "Instrument Options"="", "Check Status Callback"="", "Flags"=0, "Help"="Multi evaluation measurement results"}, {"Level"=3, "Class Only"=TRUE, "Identifier"="", "Descriptive Name"="Detected Signal Configuration", "Data Type"=enum."ViInt32", "Command"="", "Access"=enum."Read Only", "Range Table"="", "Read Callback"="", "Write Callback"="", "Range Callback"="", "Check Callback"="", "Rngtable Callback"="", "Coerce Callback"="", "Supported Models"="", "Instrument Options"="", "Check Status Callback"="", "Flags"=0, "Help"="Return the detected allocation and modulation scheme."}, {"Level"=4, "Class Only"=FALSE, "Identifier"="RSCMXPNRFR2M_ATTR_FETCH_MULTI_EVAL_MEASUREMENT_MODULATION_DETECTED_ALLOCATION_RESULTS", "Descriptive Name"="Fetch Multi Eval Measurement Modulation Detected Allocation Results", "Data Type"=enum."RawString", "Command"="FETC:NRMM:MEAS{instance}:MEV:MOD:DALL?", "Access"=enum."Read Only", "Range Table"="", "Read Callback"="", "Write Callback"="", "Range Callback"="", "Check Callback"="", "Rngtable Callback"="", "Coerce Callback"="", "Supported Models"="", "Instrument Options"="", "Check Status Callback"="", "Flags"=0, "Help"="Returns the detected allocation for the measured slot.\n\nAvailable Repeated Capabilities:\ninstance: i0, i1, i2, i3, i4, i5, i6, i7, i8, i9, i10, i11, i12, i13, i14, i15, i16, i17, i18, i19, i20, i21, i22, i23, i24, i25, i26, i27, i28, i29, i30, i31, i32\r\n\nRemote-control command(s):\nFETCh:NRMMw:MEAS<i>:MEValuation:MODulation:DALLocation?"}, {"Level"=4, "Class Only"=FALSE, "Identifier"="RSCMXPNRFR2M_ATTR_FETCH_MULTI_EVAL_MEASUREMENT_MODULATION_DETECTED_MODULATION_RESULTS", "Descriptive Name"="Fetch Multi Eval Measurement Modulation Detected Modulation Results", "Data Type"=enum."RawString", "Command"="FETC:NRMM:MEAS{instance}:MEV:MOD:DMOD?", "Access"=enum."Read Only", "Range Table"="", "Read Callback"="", "Write Callback"="", "Range Callback"="", "Check Callback"="", "Rngtable Callback"="", "Coerce Callback"="", "Supported Models"="", "Instrument Options"="", "Check Status Callback"="", "Flags"=0, "Help"="Returns the detected modulation scheme in the measured slot.\n\nAvailable Repeated Capabilities:\ninstance: i0, i1, i2, i3, i4, i5, i6, i7, i8, i9, i10, i11, i12, i13, i14, i15, i16, i17, i18, i19, i20, i21, i22, i23, i24, i25, i26, i27, i28, i29, i30, i31, i32\r\n\nRemote-control command(s):\nFETCh:NRMMw:MEAS<i>:MEValuation:MODulation:DMODulation?"}, {"Level"=4, "Class Only"=FALSE, "Identifier"="RSCMXPNRFR2M_ATTR_FETCH_MULTI_EVAL_MEASUREMENT_SEM_DALLOCATION_RESULTS", "Descriptive 
